vi "make_synth_array (SubVI).vi"(11 "Synth settings:":T1={"start volt (V)"=1.0, "stop volt (V) "=1.0, "# V Steps"=1, "start freq (Hz)"=2000.0, "stop freq (Hz) "=2000.0, "# F steps"=1, "dc offset?"=FALSE, "start DC (V)"=0.5, "stop DC (V)"=0.5, "# DC steps "=1, "Set synth\n(HP33120A)?"=FALSE, "Use arbitrary\nwaveform?"=FALSE, "Arb waveform name:"=""}) -> (3 "Tot Synth Arr":dbl[][](array[numeric]))   [LabVIEW 2018]
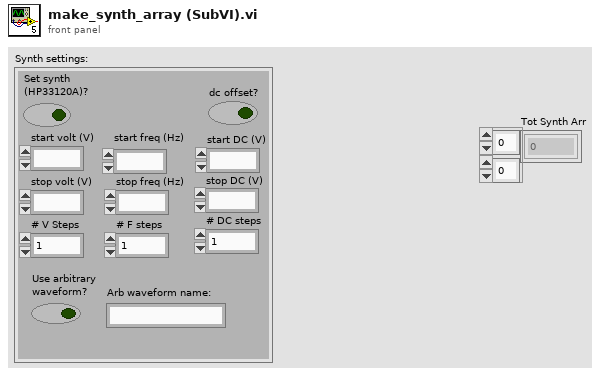
[diagram p1: front panel]
types:
  T1 = cluster{"start volt (V)":ext, "stop volt (V) ":ext, "# V Steps":i32, "start freq (Hz)":ext, "stop freq (Hz) ":ext, "# F steps":i32, "dc offset?":bool, "start DC (V)":ext, "stop DC (V)":ext, "# DC steps ":i32, "Set synth\n(HP33120A)?":bool, "Use arbitrary\nwaveform?":bool, "Arb waveform name:":string}
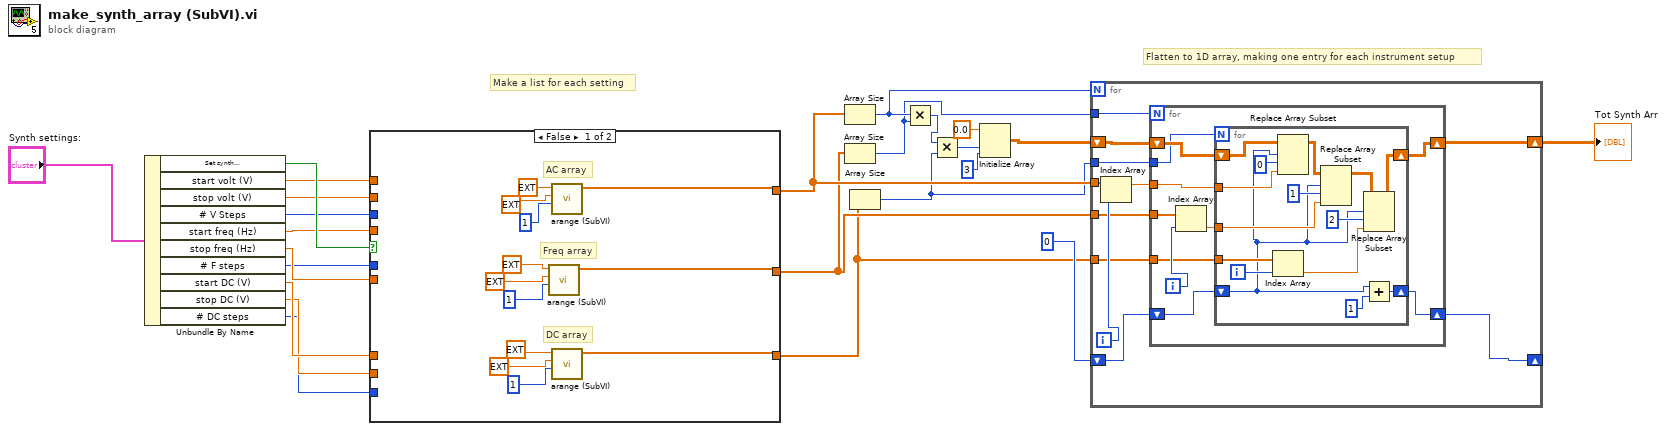
[diagram p0: block diagram]
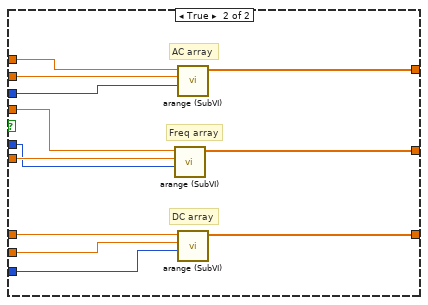
[diagram p2: hidden frame]
diagram:
  # "Make a list for each setting"
  # "Flatten to 1D array, making one entry for each instrument setup"
  n1 = Unbundle By Name("Synth settings:") -> ("Set synth\n(HP33120A)?"=w24:bool, "start volt (V)"=w23:ext, "stop volt (V)"=w22:ext, "# V Steps"=w21:i32, "start freq (Hz)"=w20:ext, "stop freq (Hz)"=w19:ext, "# F steps"=w18:i32, "start DC (V)"=w17:ext, "stop DC (V)"=w16:ext, "# DC steps"=w15:i32)
  n2 = case shown="False" w24 {
    tunnel: w23 -> [_ w48]
    tunnel: w22 -> [_ w47]
    tunnel: w21 -> [_ w46]
    tunnel: w20 -> [_ w45]
    tunnel: w19 -> [_ w44]
    tunnel: w18 -> [_ w43]
    tunnel: w17 -> [_ w42]
    tunnel: w16 -> [_ w41]
    tunnel: w15 -> [_ w40]
    tunnel: [w27 w39] -> w7
    tunnel: [w26 w38] -> w6
    tunnel: [w25 w37] -> w5
    frame False {
      # "DC array"
      # "Freq array"
      # "AC array"
      n3 = call "arange (SubVI).vi"("# Steps"=1, "stop"=ext -1.0, "start"=ext -1.0) -> ("Array"=w26:ext[])  [unwired: 8 in]
      n4 = call "arange (SubVI).vi"("# Steps"=1, "stop"=ext -1.0, "start"=ext -1.0) -> ("Array"=w27:ext[])  [unwired: 8 in]
      n5 = call "arange (SubVI).vi"("# Steps"=1, "stop"=ext -1.0, "start"=ext -1.0) -> ("Array"=w25:ext[])  [unwired: 8 in]
    }
    frame True {
      # "DC array"
      # "Freq array"
      # "AC array"
      n6 = call "arange (SubVI).vi"("# Steps"=w43, "stop"=w44, "start"=w45) -> ("Array"=w38:ext[])  [unwired: 8 in]
      n7 = call "arange (SubVI).vi"("# Steps"=w46, "stop"=w47, "start"=w48) -> ("Array"=w39:ext[])  [unwired: 8 in]
      n8 = call "arange (SubVI).vi"("# Steps"=w40, "stop"=w41, "start"=w42) -> ("Array"=w37:ext[])  [unwired: 8 in]
    }
  }
  n9 = Array Size(array=w7) -> (size(s)=w4:i32)
  n10 = Array Size(array=w6) -> (size(s)=w3:i32)
  n11 = Array Size(array=w5) -> (size(s)=w2:i32)
  n12 = Multiply(x=w4, y=w3) -> (x*y=w13:i32)
  n13 = Multiply(x=w13, y=w2) -> (x*y=w12:i32)
  n14 = Initialize Array(0.0 ("element"), w12, 3 ("dimension size")) -> (w10:dbl[][])
  n15 = for {
    N: w4 -> [_]
    shift-right: [w49] -> _
    shift-left: 0 ("disabled index (row)") -> [w50]
    shift-right: [w58] -> w8
    shift-left: w10 -> [w59]
    tunnel: w7 -> [w57]
    tunnel: w6 -> [w54]
    tunnel: w5 -> [w53]
    tunnel: w3 -> [w52]
    tunnel: w2 -> [w51]
    i -> [w55]
    n16 = Index Array(array=w57, index=w55) -> (element=w56:ext)
    n17 = for {
      N: w52 -> [_]
      tunnel: w56 -> [w67]
      tunnel: w54 -> [w66]
      tunnel: w53 -> [w63]
      tunnel: w51 -> [w62]
      shift-right: [w68] -> w58
      shift-left: w59 -> [w69]
      shift-right: [w60] -> w49
      shift-left: w50 -> [w61]
      i -> [w65]
      n18 = Index Array(array=w66, index=w65) -> (element=w64:ext)
      n19 = for {
        N: w62 -> [_]
        tunnel: w67 -> [w77]
        tunnel: w64 -> [w76]
        tunnel: w63 -> [w74]
        shift-right: [w80] -> w68
        shift-left: w69 -> [w84]
        shift-right: [w71] -> w60
        shift-left: w61 -> [w70]
        i -> [w75]
        n20 = Index Array(array=w74, index=w75) -> (element=w73:ext)
        n21 = Replace Array Subset(array=w84, new element=w77, index (row)=w70, index (col)=0 ("disabled index (col)")) -> (w82:dbl[][])
        n22 = Replace Array Subset(array=w82, new element=w76, index (row)=w70, index (col)=1 ("disabled index (col)")) -> (w81:dbl[][])
        n23 = Replace Array Subset(array=w81, new element=w73, index (row)=w70, index (col)=2 ("disabled index (col)")) -> (w80:dbl[][])
        n24 = Add(x=w70, y=1) -> (x+y=w71:i32)
      }
    }
  }
  "Tot Synth Arr" <- w8
